vi "Write UID.vi"(5 "UID":i32, 9 "GObject in":refnum<class "GObject.lvclass">) -> (3 "GObject out":refnum<class "GObject.lvclass">)   [LabVIEW 2014, in "Raspberry Pi Compatible Compiler for LabVIEW.lvlib" / "GObject.lvclass"]
uses:
  GObject.lvclass
  GObject.lvclass/GObject.ctl
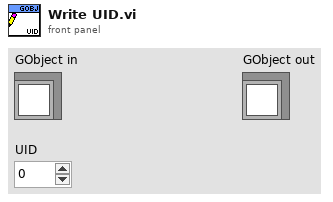
[diagram p1: front panel]
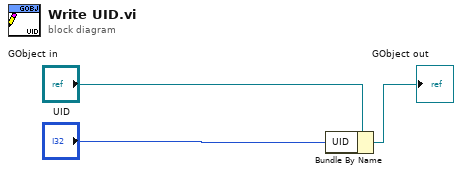
[diagram p0: block diagram]
diagram:
  n1 = Bundle By Name(cluster="GObject in", "UID"="UID") -> (→"GObject out":refnum<class "GObject.lvclass">)
